vi "CRYUpdate Calibration Information.vi"(8 "From Hardware?":bool, 9 "Hardware Channel Array":T1[](array[typedef]) {"Coupling" items=["Default"=-1, "RSE"=10083, "NRSE"=10078, "Differential"=10106, "Pseudodifferential"=12529]; "term config" items=["Default"=-1, "RSE"=10083, "NRSE"=10078, "Differential"=10106, "Pseudodifferential"=12529]; "Anti-aliasing Factor (%fs)" format="%.2f"}, 10 "O_Name In":string[][](array[string]), 11 "I_Name In":string[][](array[string])) -> (3 "Detail Information Out":string[][](array[string]))   [LabVIEW 2013]
uses:
  Typedef Control/CRYHardware Channel Info.ctl
  CRYProject/CRYProject Editor Global.vi
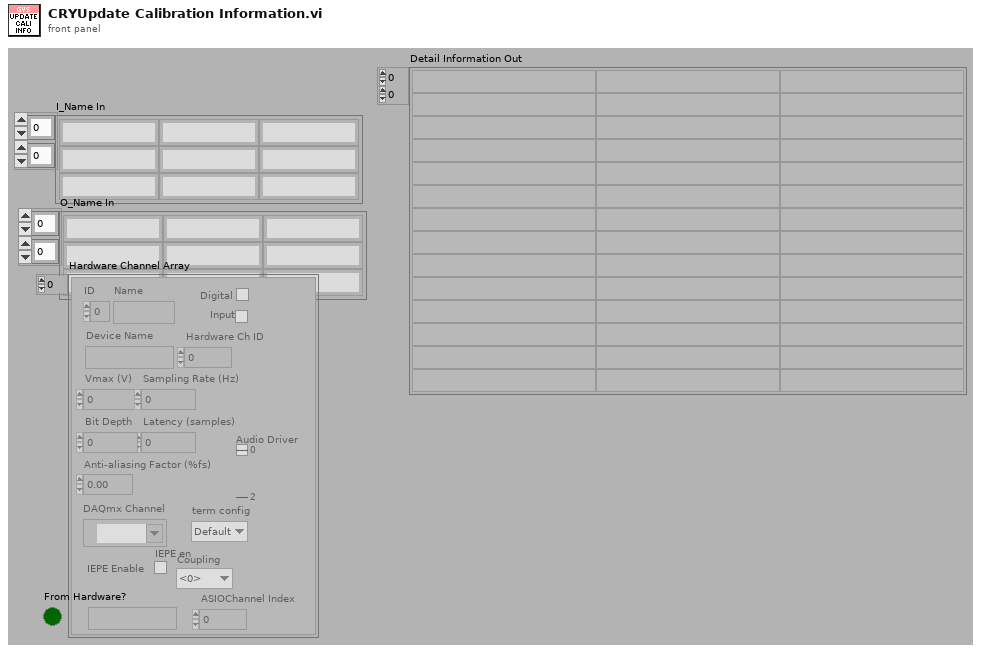
[diagram p1: front panel]
types:
  T1 = typedef "CRYHardware Channel Info.ctl" = cluster{"ID":i32, "Name":string, "Digital":bool, "Input":bool, "Device Name":string, "Hardware Ch ID":u8, "Vmax (V)":dbl, "Latency (samples)":dbl, "Sampling Rate (Hz)":u32, "Bit Depth":u32, "Anti-aliasing Factor (%fs)":sgl, "DAQmx Channel":tag, "term config":i32, "Coupling":i32, "IEPE en":bool, "ASIOChannel Name":string, "Audio Driver":u16, "ASIOChannel Index":u8}
  T2 = typedef "CRYCalibration All Cluster.ctl" = cluster{"Calibration 2D":T3[], "Help":string, "Tab Value":i32, "Input Signal Type":string, "Output Signal Type":string}
  T3 = typedef "CRYCalibration 2DCluster.ctl" = cluster{"Calibration":T4, "Corr Curve":T5, "EQ Curve":T5, "Sens Curve":T5}
  T4 = typedef "CRYCalibration Cluster.ctl" = cluster{"Calibration Step Name":string, "Device":string, "Correction Curve Name":string, "Equalization Curve Name":string, "Sensitivity Curve Name":string, "Corr Folder and File":string, "EQ Folder and File":string, "Sens Folder and File":string, "Corr Step size":u16, "EQ Step size":u16, "Input":bool, "Last Cal Date (sec)":timestamp, "Cha Name":string, "Corr Curve Found":bool, "EQ Curve Found":bool, "Sens Curve Found":bool, "Signal Type":string, "Calibrated Device":string, "Hz":u32}
  T5 = typedef "CRYData Cluster.ctl" = cluster{"Name":string, "Curve":cluster{"x":dbl, "y":dbl, "z":dbl}[], "X data":u16, "Y data":u16, "Z data":u16, "X axis":u16, "Y axis":u16, "Z axis":u16, "X unit":string, "Y unit":string, "Z unit":string, "X dB ref":dbl, "Y dB ref":dbl, "Z dB ref":dbl, "single val":bool, "protected":bool, "display X":bool, "display Y":bool, "display Z":bool, "Test Info":string, "Step No.":i32, "Plot Settings":cluster{"Color":u32, "Interpolation":u8, "Point Style":u8, "Line Style":u8, "Point Color":u32, "Line Width":u8, "Bar Plot Style":u8, "Fill To":i16}, "AutoProtect":bool}
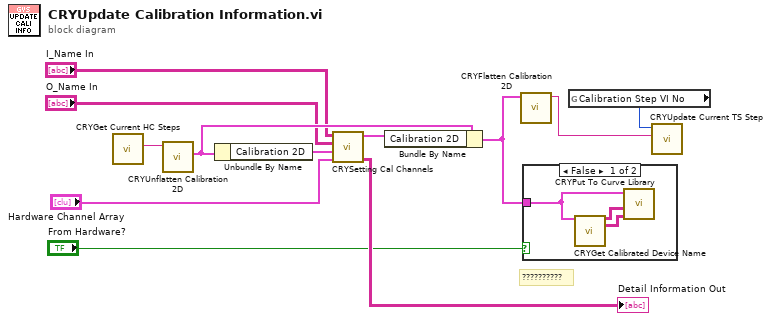
[diagram p0: block diagram]
diagram:
  # "??????????"
  n1 = call "CRYGet Current HC Steps.vi"() -> ("Calibration setup flattened Out"=w12:string)  [unwired: 11 out]
  n2 = call "CRYUnflatten Calibration 2D.vi"("Flattened Calibration"=w12) -> ("Calibration Step Out"=w10:T2)  [unwired: 10 out]
  n3 = Unbundle By Name(w10) -> ("Calibration 2D"=w11:T3[])
  n4 = call "CRYSetting Cal Channels.vi"("Hardware Channel Array"="Hardware Channel Array", "Calibration 2D Array"=w11, "O_Name In"="O_Name In", "I_Name In"="I_Name In") -> ("Detail Information Out"=→"Detail Information Out":string[][], "Calibration Out"=w9:T3[])  [unwired: 1 in, 5 out]
  n5 = Bundle By Name(cluster=w10, "Calibration 2D"=w9) -> (w4:T2)
  n6 = call "CRYFlatten Calibration 2D.vi"("Calibration All Cluster"=w4) -> ("Calibration flattened"=w3:string)  [unwired: 10 in]
  n7 = case shown="False" "From Hardware?" {
    tunnel: w4 -> [w15 _]
    frame False {
      n8 = call "CRYGet Calibrated Device Name.vi"("Calibration"=w15) -> ("I_Name Out(Input Calibrated Name Out)"=w14:string[][], "O_Name Out(Output Calibrated Name Out)"=w13:string[][])  [unwired: 7 in, 6 out]
      n9 = call "CRYPut To Curve Library.vi"("O_Calibrated Device Name In"=w13, "I_Calibrated Device Name In"=w14, "Calibration Step Cluster"=w15) -> ()  [unwired: 3 in, 6 out]
    }
    frame True {
    }
  }
  n10 = global read "CRYProject Editor Global.vi" "Calibration Step VI No"() -> (w1:i32)
  n11 = call "CRYUpdate Current TS Step.vi"("setup flattened"=w3, "step index"=w1) -> ()  [unwired: 10 out]
